vi "Create FPGA Reference (iSUB) (SubVI).vi"() -> (3 "FPGA REF (iSUB)":T1)   [LabVIEW 2015]
uses:
  Controls (HOST)/FPGA REF (iSUB).ctl
  <vilib>/FPGAPlugInAG/PCIe-1473R-LX110/niLvFpga_Open_PCIe-1473R-LX110.vi
  <vilib>/rvi/interface/common/dynamic/niFpgaDynamicAddResources.vi
  <vilib>/FPGAPlugInAG/Dynamic/niLvFpga_Reset_Dynamic.vi
  <vilib>/rvi/interface/nirviOpenFPGA/nirviOpenFPGA.xnode
  FPGA Bitfiles/IMAQ (iSUB).lvbitx
  <vilib>/rvi/interface/nirviMethod/nirviMethod.xnode
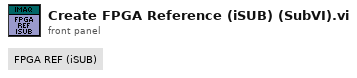
[diagram p1: front panel]
types:
  T1 = typedef "FPGA REF (iSUB).ctl" = refnum<k20>
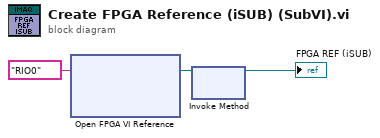
[diagram p0: block diagram]
diagram:
  n1 = xnode "Open FPGA VI Reference"("resource name"=tag "RIO0") -> ("FPGA VI Reference Out"=w2:refnum<k20>)  [unwired: 1 in, 1 out]
  n2 = xnode "Invoke Method"("FPGA VI Reference In"=w2) -> ("FPGA VI Reference Out"=→"FPGA REF (iSUB)":refnum<k20>)  [unwired: 1 in, 1 out]
